vi "Teleop.vi"(10 "Match Info":T1={"Autonomous Elapsed Seconds"=0.0, "TeleOp Elapsed Seconds"=0.0, "Disabled Elapsed Seconds"=0.0, "Visited Autonomous"=FALSE, "Visited TeleOp"=FALSE, "Visited Disabled"=FALSE, "Autonomous Settings"={"Autonomous Style"=enum."Independent", "VI Refnum"=refnum}}, 11 "Call Context":T2) -> ()   [LabVIEW 2014]
doc: "This VI is called for each TeleOp packet received from the DS where the robot is not disabled. It is often used to read from the joysticks and update I/O or to update setpoints for timed control loops. It should complete and return within 20 milliseconds or it may miss DS packets."
uses:
  <vilib>/Rock Robotics/WPI/DriverStation/WPI_DriverStationDerivedRobotMode.ctl
  <vilib>/Rock Robotics/WPI/DriverStation/WPI_DriverStationMatch Info.ctl
  <vilib>/Rock Robotics/WPI/RobotDrive/WPI_RobotDriveGetSetRefNum.vi
  <vilib>/Rock Robotics/WPI/Joystick/WPI_JoystickGetSetRefNum.vi
  Robot Global Data.vi
  <vilib>/Rock Robotics/Network Tables/SD Write Boolean Array.vi
  <vilib>/Rock Robotics/Network Tables/SD Write Numeric Array.vi
  <vilib>/Rock Robotics/Network Tables/SD Read Number.vi
  <vilib>/Rock Robotics/Network Tables/SD Write Boolean.vi
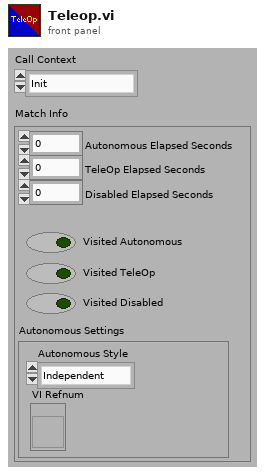
[diagram p1: front panel]
types:
  T1 = typedef "WPI_DriverStationMatch Info.ctl" = cluster{"Autonomous Elapsed Seconds":dbl, "TeleOp Elapsed Seconds":dbl, "Disabled Elapsed Seconds":dbl, "Visited Autonomous":bool, "Visited TeleOp":bool, "Visited Disabled":bool, "Autonomous Settings":cluster{"Autonomous Style":enum16{"Iterative", "Independent"}, "VI Refnum":refnum<vi>}}
  T2 = typedef "WPI_DriverStationDerivedRobotMode.ctl" = enum16{"Init", "Execute", "Stop"}
  T3 = typedef "WPI_JoystickDevRef.ctl" = cluster{"Device":T4}
  T4 = typedef "WPI_JoystickDeviceEnum.ctl" = enum16{"USB 0", "USB 1", "USB 2", "USB 3", "USB 4", "USB 5"}
  T5 = cluster{"POVs[0]":i16, "POVs[1]":i16, "POVs[2]":i16, "POVs[3]":i16, "POVs[4]":i16, "POVs[5]":i16, "POVs[6]":i16, "POVs[7]":i16, "POVs[8]":i16}
  T6 = cluster{"TopLeft":bool, "TopCenter":bool, "TopRight":bool, "MiddleRight":bool, "MiddleLeft":bool, "MiddleCenter":bool, "BottomRight":bool, "BottomLeft":bool, "BottomCenter":bool, "Top":bool, "Middle":bool, "Bottom":bool, "Left":bool, "Center":bool, "Right":bool}
  T7 = cluster{"Axes[0]":dbl, "Axes[1]":dbl, "Axes[2]":dbl, "Axes[3]":dbl, "Axes[4]":dbl, "Axes[5]":dbl, "Axes[6]":dbl, "Axes[7]":dbl, "Axes[8]":dbl}
  T8 = cluster{"Buttons[0]":bool, "Buttons[1]":bool, "Buttons[2]":bool, "Buttons[3]":bool, "Buttons[4]":bool, "Buttons[5]":bool, "Buttons[6]":bool, "Buttons[7]":bool, "Buttons[8]":bool, "Buttons[9]":bool, "Buttons[10]":bool, "Buttons[11]":bool, "Buttons[12]":bool, "Buttons[13]":bool, "Buttons[14]":bool, "Buttons[15]":bool}
  T9 = cluster{"Buttons[0]":bool, "Buttons[1]":bool, "Buttons[2]":bool, "Buttons[3]":bool, "Buttons[4]":bool, "Buttons[5]":bool, "Buttons[6]":bool, "Buttons[7]":bool, "Buttons[8]":bool}
  T10 = typedef "WPI_RobotDriveDevRef.ctl" = cluster{"DevStatus":errorcluster, "Motors[]":T11[], "Square Inputs":bool, "Max Output":dbl}
  T11 = typedef "WPI_MotorControlDeviceRef.ctl" = cluster{"DeviceStatus":errorcluster, "Type":T12, "PWM":cluster{"Controller":T13, "PWM Channel":T14, "DeadBand":T15}, "CAN":cluster{"Device Number":u8, "Control Mode":T16, "Semaphore":T17, "Max Vout":dbl, "TalonSRX Control Mode":T18}, "Invert":bool, "TransformRef":T19, "InvTransformRef":T19}
  T12 = typedef "WPI_MotorControlType.ctl" = enum16{"PWM", "CAN", "CANTalonSRX"}
  T13 = typedef "FPGA_TypedefDigitalModule.ctl" = enum16{"Controller 1"}
  T14 = typedef "FPGA_DIOPWMChannel.ctl" = enum8{"PWM 0", "PWM 1", "PWM 2", "PWM 3", "PWM 4", "PWM 5", "PWM 6", "PWM 7", "PWM 8", "PWM 9", "PWM MXP 0", "PWM MXP 1", "PWM MXP 2", "PWM MXP 3", "PWM MXP 4", "PWM MXP 5", "PWM MXP 6", "PWM MXP 7", "PWM MXP 8", "PWM MXP 9", "Invalid"}
  T15 = typedef "WPI_PWMDeadband.ctl" = cluster{"Name":string, "maxPositivePwm":i32, "minPositivePwm":i32, "centerPwm":i32, "maxNegativePwm":i32, "minNegativePwm":i32, "angularRange":u16}
  T16 = typedef "WPI_CANJaguar_ControlMode.ctl" = enum8{"Percent VBus", "Current", "Speed", "Position", "Voltage"}
  T17 = typedef "Semaphore RefNum" = refnum<k1>
  T18 = typedef "WPI_CANTalonSRX_APIControlMode.ctl" = enum8{"Percent VBus", "Speed", "Position", "Slave", "Unchanged / Invalid"}
  T19 = typedef "WPI_PWMTransform_ConPane.ctl" = refnum<vi>
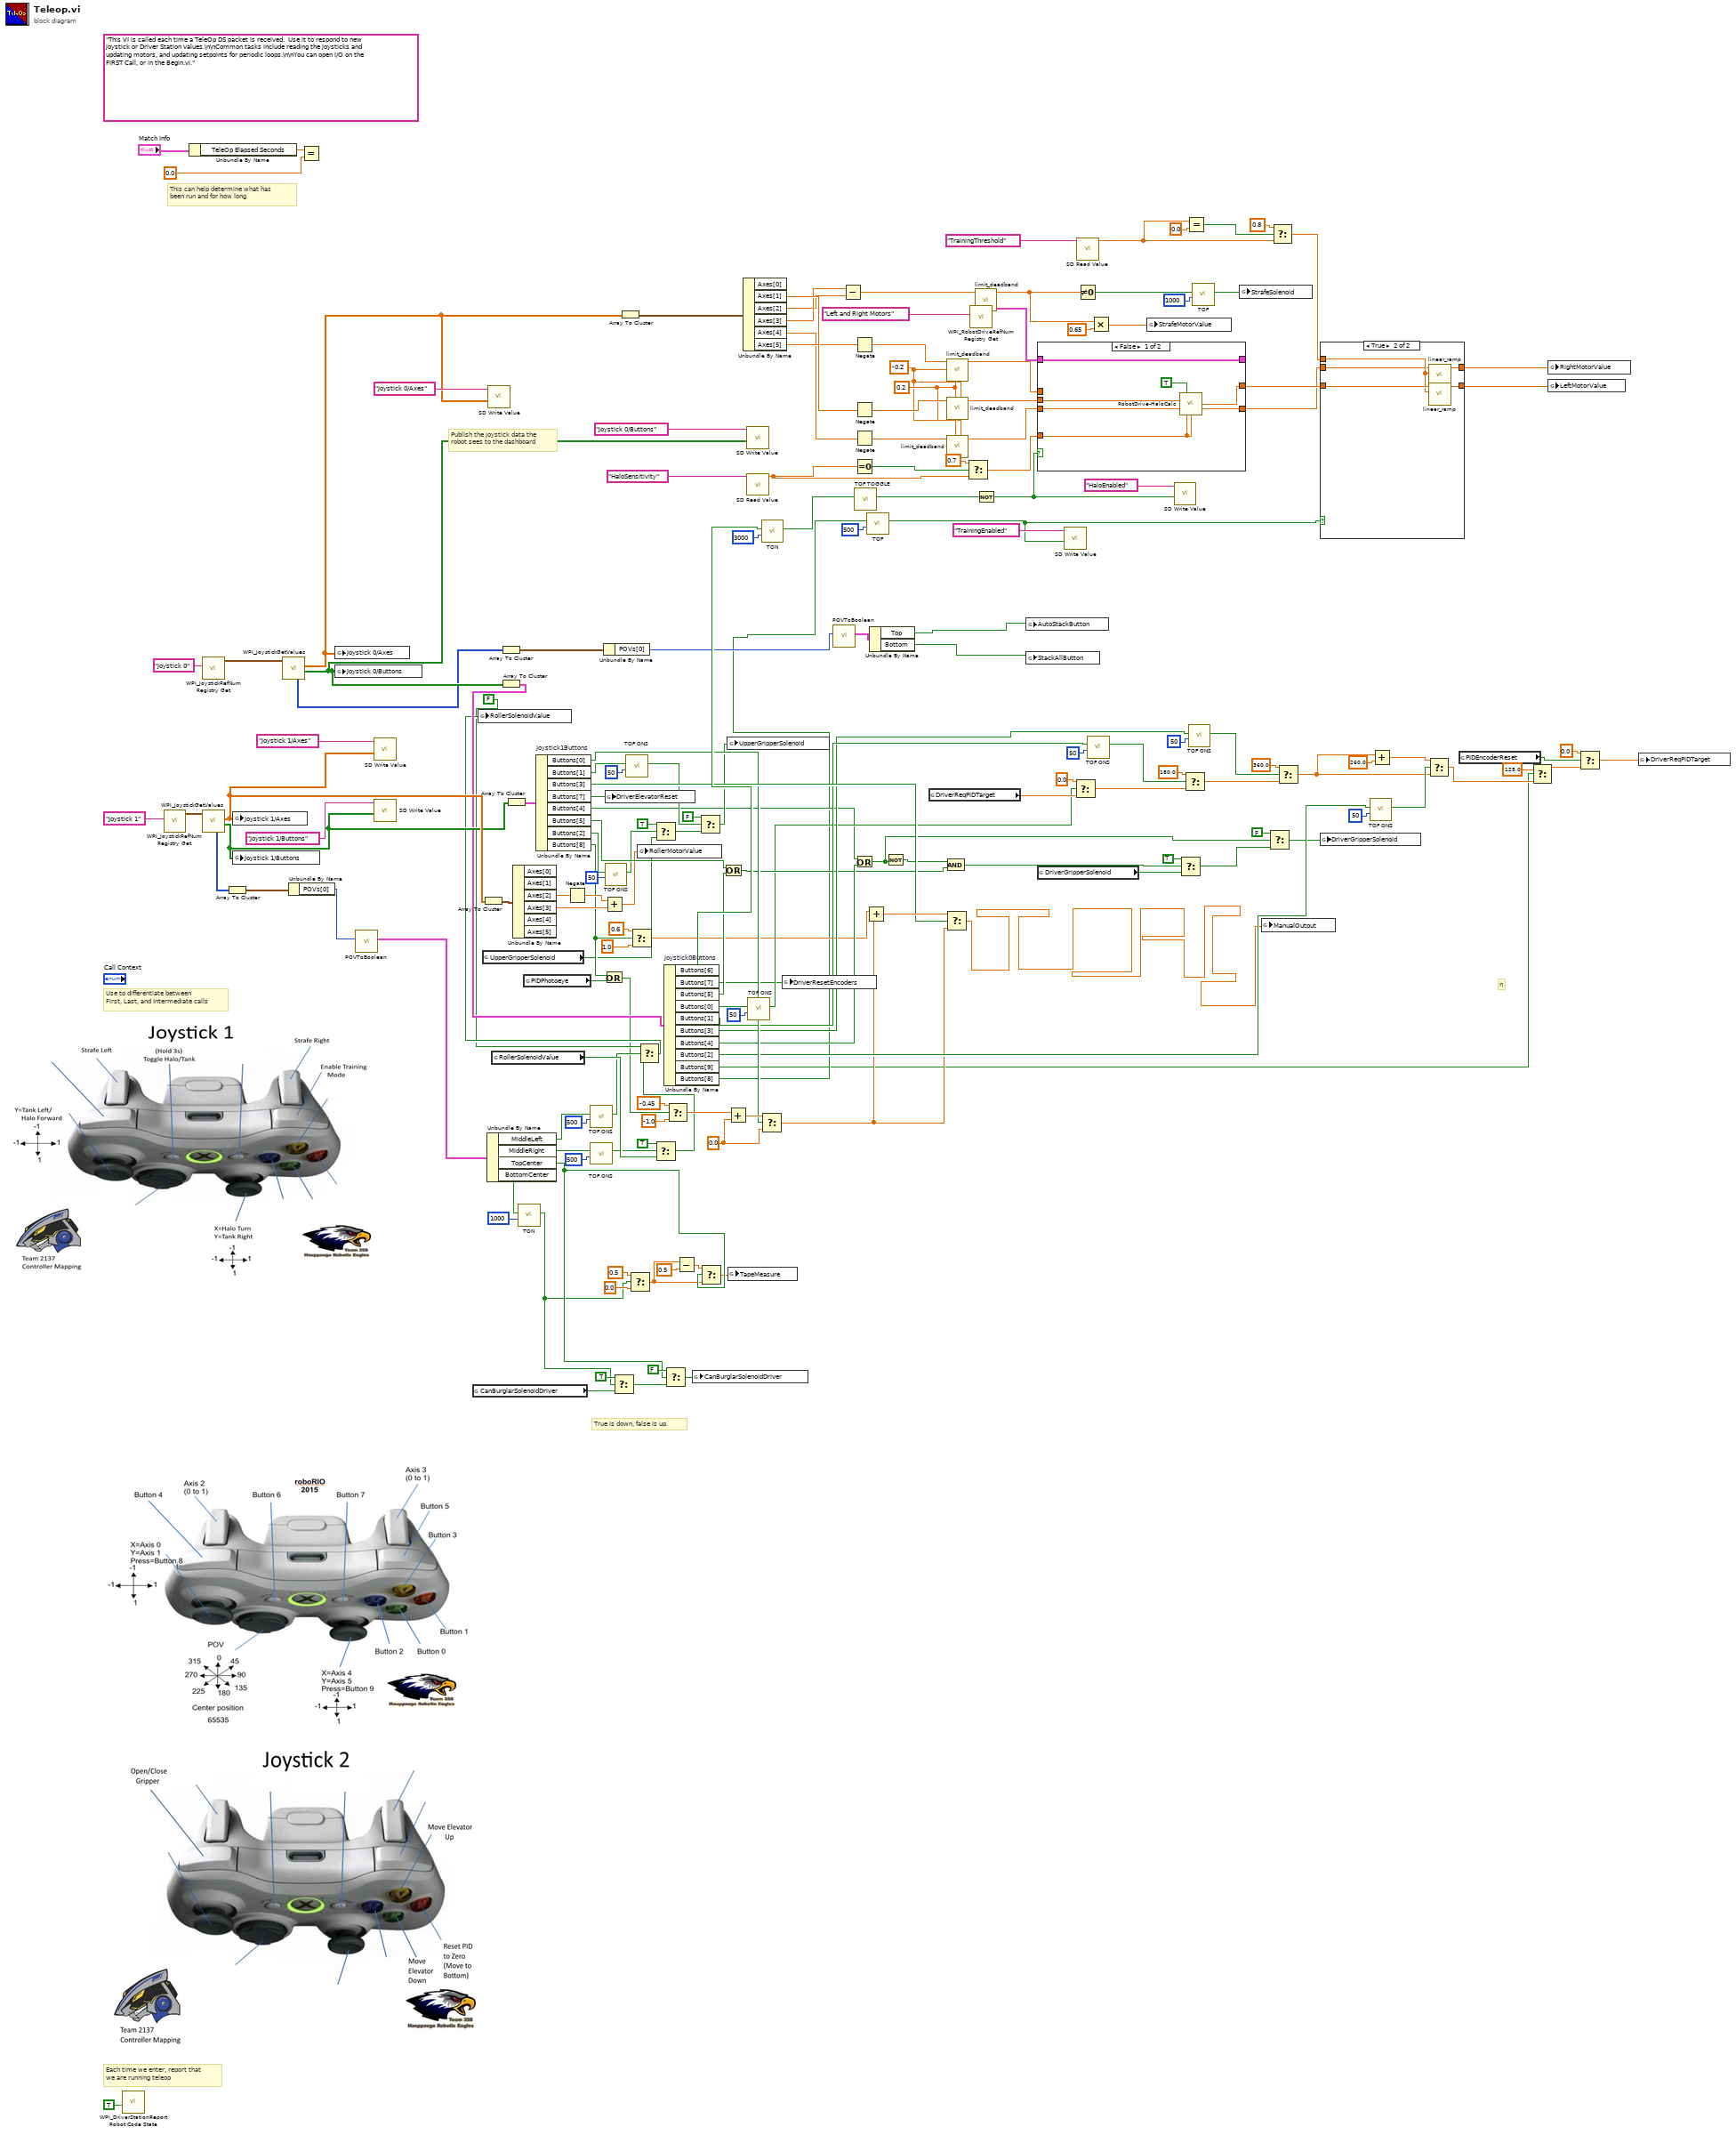
[diagram p0: block diagram]
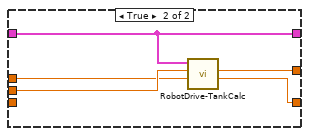
[diagram p3: hidden frame]
diagram:
  w78 = -0.2
  w79 = 0.2
  w141 = 0.0
  (unwired) "This VI is called each time a TeleOp DS packet is received.  Use it to respond to new joystick or Driver Station values.\n\nCommon tasks include reading the joysticks and updating motors, and updating setpoints for periodic loops.\n\nYou can open I/O on the FIRST Call, or in the Begin.vi."
  # "n"
  # "True is down, false is up."
  # "Publish the joystick data the\nrobot sees to the dashboard"
  # "Each time we enter, report that\nwe are running teleop"
  # "Use to differentiate between\nFirst, Last, and Intermediate calls"
  # "This can help determine what has\nbeen run and for how long"
  n1 = call <vilib>:"WPI_DriverStationReport Robot Code State.vi"("TeleOp"=TRUE ("Autonomous")) -> ()  [unwired: 10 in, 1 out]
  n2 = call <vilib>:"WPI_JoystickRefNum Registry Get.vi"("refnum name"="Joystick 1") -> ("JoystickDevRef"=w152:T3)  [unwired: 1 in, 9 out]
  n3 = Unbundle By Name("Match Info") -> ("TeleOp Elapsed Seconds"=w144:dbl)
  n4 = call <vilib>:"WPI_JoystickRefNum Registry Get.vi"("refnum name"="Joystick 0") -> ("JoystickDevRef"=w174:T3)  [unwired: 1 in, 9 out]
  n5 = call <vilib>:"WPI_JoystickGetValues.vi"("JoystickDevRef"=w152) -> ("Buttons"=w147:bool[], "Axes"=w148:dbl[], "POVs"=w58:i16[])  [unwired: 6 in, 2 out]
  n6 = Array To Cluster(array=w58) -> (cluster=w57:T5)
  n7 = global write "Robot Global Data.vi" "Joystick 1/Axes"(w148) -> ()
  n8 = global write "Robot Global Data.vi" "Joystick 1/Buttons"(w147) -> ()
  n9 = call <vilib>:"WPI_JoystickGetValues.vi"("JoystickDevRef"=w174) -> ("Buttons"=w145:bool[], "Axes"=w146:dbl[], "POVs"=w102:i16[])  [unwired: 6 in, 2 out]
  n10 = Unbundle By Name(w57) -> ("POVs[0]"=w56:i16)
  n11 = Equal?(x=w144, y=0.0) -> ()  [unwired: 1 out]
  n12 = global write "Robot Global Data.vi" "Joystick 0/Axes"(w146) -> ()
  n13 = global write "Robot Global Data.vi" "Joystick 0/Buttons"(w145) -> ()
  n14 = call "POVToBoolean.vi"("Input"=w56) -> ("Output"=w55:T6)  [unwired: 10 in]
  n15 = call-poly <vilib>:"SD Write Value.vi"("Numeric Array"=w148, "Name"="Joystick 1/Axes") -> ()  [unwired: 8 in, 2 out]
  n16 = call-poly <vilib>:"SD Write Value.vi"("Boolean Array"=w147, "Name"="Joystick 1/Buttons") -> ()  [unwired: 8 in, 2 out]
  n17 = global read "Robot Global Data.vi" "CanBurglarSolenoidDriver"() -> (w19:bool)
  n18 = Array To Cluster(array=w148) -> (cluster=w149:T7)
  n19 = global read "Robot Global Data.vi" "UpperGripperSolenoid"() -> (w22:bool)
  n20 = Unbundle By Name(w55) -> ("MiddleLeft"=w53:bool, "MiddleRight"=w54:bool, "TopCenter"=w16:bool, "BottomCenter"=w2:bool)
  n21 = call-poly <vilib>:"SD Write Value.vi"("Numeric Array"=w146, "Name"="Joystick 0/Axes") -> ()  [unwired: 8 in, 2 out]
  n22 = global read "Robot Global Data.vi" "RollerSolenoidValue"() -> (w50:bool)
  n23 = Array To Cluster(array=w102) -> (cluster=w103:T5)
  n24 = Array To Cluster(array=w145) -> (cluster=w77:T8)
  n25 = Array To Cluster(array=w147) -> (cluster=w142:T9)
  n26 = Unbundle By Name(w149) -> ("Axes[2]"=w63:dbl, "Axes[3]"=w44:dbl)  [unwired: 4 out]
  n27 = call "TON.vi"("Delay (ms)"=u32 1000, "Input"=w2) -> ("Output"=w3:bool)  [unwired: 9 in]
  n28 = global read "Robot Global Data.vi" "PIDPhotoeye"() -> (w89:bool)
  n29 = Unbundle By Name "Joystick1Buttons"(w142) -> ("Buttons[0]"=w128:bool, "Buttons[1]"=w35:bool, "Buttons[3]"=w129:bool, "Buttons[7]"=w107:bool, "Buttons[4]"=w27:bool, "Buttons[5]"=w75:bool, "Buttons[2]"=w33:bool, "Buttons[8]"=w38:bool)
  n30 = Negate(x=w63) -> (-x=w45:dbl)
  n31 = call "TOF ONS.vi"("Delay (ms)"=u32 500, "Input"=w53) -> ("Output"=w46:bool)  [unwired: 9 in]
  n32 = call "TOF ONS.vi"("Delay (ms)"=u32 500, "Input"=w54) -> ("Output"=w48:bool)  [unwired: 9 in]
  n33 = Unbundle By Name(w103) -> ("POVs[0]"=w42:i16)
  n34 = Add(x=w45, y=w44) -> (x+y=w62:dbl)
  n35 = Or(x=w38, y=w89) -> (x .or. y?=w43:bool)
  n36 = global write "Robot Global Data.vi" "DriverElevatorReset"(w107) -> ()
  n37 = call "TOF ONS.vi"("Delay (ms)"=u32 50, "Input"=w33) -> ("Output"=w28:bool)  [unwired: 9 in]
  n38 = Select(t=TRUE, s=w3, f=w19) -> (s? t:f=w20:bool)
  n39 = Array To Cluster(array=w146) -> (cluster=w170:T7)
  n40 = call "TOF ONS.vi"("Delay (ms)"=u32 50, "Input"=w35) -> ("Output"=w30:bool)  [unwired: 9 in]
  n41 = Select(t=0.5 ("y"), s=w3, f=0.0) -> (s? t:f=w10:dbl)
  n42 = Select(t=0.6, s=w38, f=1.0 ("x")) -> (s? t:f=w37:dbl)
  n43 = global write "Robot Global Data.vi" "RollerMotorValue"(w62) -> ()
  n44 = Select(t=TRUE, s=w28, f=w22) -> (s? t:f=w29:bool)
  n45 = Select(t=TRUE, s=w48, f=w50) -> (s? t:f=w51:bool)
  n46 = Select(t=FALSE, s=w46, f=w51) -> (s? t:f=w52:bool)
  n47 = global write "Robot Global Data.vi" "RollerSolenoidValue"(w52) -> ()
  n48 = Unbundle By Name "Joystick0Buttons"(w77) -> ("Buttons[6]"=w158:bool, "Buttons[7]"=w9:bool, "Buttons[5]"=w76:bool, "Buttons[0]"=w122:bool, "Buttons[1]"=w125:bool, "Buttons[3]"=w118:bool, "Buttons[4]"=w74:bool, "Buttons[2]"=w108:bool, "Buttons[9]"=w5:bool, "Buttons[8]"=w8:bool)
  n49 = Select(t=FALSE, s=w16, f=w20) -> (s? t:f=w21:bool)
  n50 = Select(t=-0.45, s=w43, f=-1.0 ("x")) -> (s? t:f=w86:dbl)
  n51 = Subtract(x=w10, y=0.5) -> (x-y=w14:dbl)
  n52 = global write "Robot Global Data.vi" "CanBurglarSolenoidDriver"(w21) -> ()
  n53 = Select(t=FALSE, s=w30, f=w29) -> (s? t:f=w31:bool)
  n54 = Select(t=w14, s=w16, f=w10) -> (s? t:f=w15:dbl)
  n55 = Or(x=w75, y=w76) -> (x .or. y?=w67:bool)
  n56 = global write "Robot Global Data.vi" "UpperGripperSolenoid"(w31) -> ()
  n57 = Add(x=w86, y=w141) -> (x+y=w140:dbl)
  n58 = global write "Robot Global Data.vi" "TapeMeasure"(w15) -> ()
  n59 = Unbundle By Name(w170) -> ("Axes[1]"=w169:dbl, "Axes[2]"=w163:dbl, "Axes[3]"=w164:dbl, "Axes[4]"=w155:dbl, "Axes[5]"=w167:dbl)  [unwired: 1 out]
  n60 = call-poly <vilib>:"SD Write Value.vi"("Boolean Array"=w145, "Name"="Joystick 0/Buttons") -> ()  [unwired: 8 in, 2 out]
  n61 = call-poly <vilib>:"SD Read Value.vi"("Name"="HaloSensitivity") -> ("Numeric"=w99:dbl)  [unwired: 8 in, 2 out]
  n62 = call "TOF ONS.vi"("Delay (ms)"=u32 50, "Input"=w122) -> ("Output"=w61:bool)  [unwired: 9 in]
  n63 = Select(t=w140, s=w128, f=w141) -> (s? t:f=w65:dbl)
  n64 = call "TON.vi"("Delay (ms)"=u32 3000, "Input"=w158) -> ("Output"=w159:bool)  [unwired: 9 in]
  n65 = global write "Robot Global Data.vi" "DriverResetEncoders"(w9) -> ()
  n66 = call "POVToBoolean.vi"("Input"=w42) -> ("Output"=w41:T6)  [unwired: 10 in]
  n67 = Subtract(x=w164, y=w163) -> (x-y=w165:dbl)
  n68 = Negate(x=w167) -> (-x=w166:dbl)
  n69 = Negate(x=w169) -> (-x=w168:dbl)
  n70 = Negate(x=w155) -> (-x=w156:dbl)
  n71 = Equal To 0?(x=w99) -> (x = 0?=w101:bool)
  n72 = Or(x=w27, y=w74) -> (x .or. y?=w36:bool)
  n73 = call "TOF TOGGLE.vi"("Input"=w159) -> ("Output"=w130:bool)  [unwired: 10 in]
  n74 = Add(x=w37, y=w65) -> (x+y=w139:dbl)
  n75 = call "TOF.vi"("Delay (ms)"=u32 500, "Input"=w8) -> ("Output"=w91:bool)  [unwired: 9 in]
  n76 = Unbundle By Name(w41) -> ("Top"=w25:bool, "Bottom"=w24:bool)
  n77 = Not(x=w36) -> (.not. x?=w66:bool)
  n78 = global read "Robot Global Data.vi" "DriverReqPIDTarget"() -> (w90:dbl)
  n79 = Select(t=w139, s=w129, f=w65) -> (s? t:f=w64:dbl)
  n80 = call "limit_deadband.vi"("lower limit"=w78, "upper limit"=w79, "Val"=w166) -> ("Val Out"=w160:dbl)  [unwired: 8 in]
  n81 = call "limit_deadband.vi"("lower limit"=w78, "upper limit"=w79, "Val"=w168) -> ("Val Out"=w161:dbl)  [unwired: 8 in]
  n82 = call "limit_deadband.vi"("lower limit"=w78, "upper limit"=w79, "Val"=w156) -> ("Val Out"=w154:dbl)  [unwired: 8 in]
  n83 = Compound Arithmetic op=AND(w66, w67) -> (w73:bool)
  n84 = Select(t=0.7, s=w101, f=w99) -> (s? t:f=w98:dbl)
  n85 = call <vilib>:"WPI_RobotDriveRefNum Registry Get.vi"("refnum name"="Left and Right Motors") -> ("RobotDriveDevRef"=w162:T10)  [unwired: 1 in, 9 out]
  n86 = call "limit_deadband.vi"("Val"=w165) -> ("Val Out"=w80:dbl)  [unwired: 10 in]
  n87 = Not(x=w130) -> (.not. x?=w114:bool)
  n88 = global write "Robot Global Data.vi" "AutoStackButton"(w25) -> ()
  n89 = global write "Robot Global Data.vi" "StackAllButton"(w24) -> ()
  n90 = case shown="False" w114 {
    tunnel: w162 -> [w181 w185]
    tunnel: [w184 w189] -> w136
    tunnel: [w183 w188] -> w133
    tunnel: w161 -> [w182 w187]
    tunnel: w160 -> [_ w186]
    tunnel: w98 -> [w178 _]
    tunnel: [w181 w185] -> _
    tunnel: w154 -> [w179 _]
    frame False {
      n91 = call "RobotDrive-HaloCalc.vi"("QwikTurnButton"=TRUE, "Left axis value"=w182, "Right axis value"=w179, "Sensitivity"=w178, "QuikTurn Sensitivity"=w178) -> ("Left Output"=w184:dbl, "Right Output"=w183:dbl)  [unwired: 9 in]
    }
    frame True {
      n92 = call "RobotDrive-TankCalc.vi"("Right axis value"=w186, "Left axis value"=w187, "RobotDriveDevRef"=w185) -> ("Right motor value"=w188:dbl, "Left motor value"=w189:dbl)  [unwired: 7 in]
    }
  }
  n93 = global read "Robot Global Data.vi" "DriverGripperSolenoid"() -> (w72:bool)
  n94 = call-poly <vilib>:"SD Write Value.vi"("Boolean"=w91, "Name"="TrainingEnabled") -> ()  [unwired: 8 in, 2 out]
  n95 = Select(t=0.0, s=w61, f=w90) -> (s? t:f=w126:dbl)
  n96 = call-poly <vilib>:"SD Read Value.vi"("Name"="TrainingThreshold") -> ("Numeric"=w94:dbl)  [unwired: 8 in, 2 out]
  n97 = Not Equal To 0?(x=w80) -> (x != 0?=w83:bool)
  n98 = call "TOF ONS.vi"("Delay (ms)"=u32 50, "Input"=w125) -> ("Output"=w123:bool)  [unwired: 9 in]
  n99 = Multiply(x=w80, y=0.65) -> (x*y=w85:dbl)
  n100 = global write "Robot Global Data.vi" "StrafeMotorValue"(w85) -> ()
  n101 = call-poly <vilib>:"SD Write Value.vi"("Boolean"=w114, "Name"="HaloEnabled") -> ()  [unwired: 8 in, 2 out]
  n102 = Select(t=TRUE, s=w73, f=w72) -> (s? t:f=w70:bool)
  n103 = Select(t=180.0, s=w123, f=w126) -> (s? t:f=w117:dbl)
  n104 = Equal?(x=w94, y=0.0) -> (x = y?=w96:bool)
  n105 = call "TOF ONS.vi"("Delay (ms)"=u32 50, "Input"=w118) -> ("Output"=w115:bool)  [unwired: 9 in]
  n106 = call "TOF.vi"("Delay (ms)"=u32 1000, "Input"=w83) -> ("Output"=w81:bool)  [unwired: 9 in]
  n107 = global write "Robot Global Data.vi" "StrafeSolenoid"(w81) -> ()
  n108 = global write "Robot Global Data.vi" "ManualOutput"(w64) -> ()
  n109 = Select(t=FALSE, s=w36, f=w70) -> (s? t:f=w68:bool)
  n110 = Select(t=0.8, s=w96, f=w94) -> (s? t:f=w93:dbl)
  n111 = Select(t=360.0, s=w115, f=w117) -> (s? t:f=w110:dbl)
  n112 = case shown="True" w91 {
    tunnel: [w191 w195] -> w135
    tunnel: w136 -> [w191 w196]
    tunnel: [w190 w192] -> w134
    tunnel: w133 -> [w190 w193]
    tunnel: w93 -> [_ w194]
    frame False {
    }
    frame True {
      n113 = call "linear_ramp.vi"("filter const (dx/dt)"=w194, "input"=w193) -> ("output"=w192:dbl)  [unwired: 9 in]
      n114 = call "linear_ramp.vi"("filter const (dx/dt)"=w194, "input"=w196) -> ("output"=w195:dbl)  [unwired: 9 in]
    }
  }
  n115 = global write "Robot Global Data.vi" "DriverGripperSolenoid"(w68) -> ()
  n116 = call "TOF ONS.vi"("Delay (ms)"=u32 50, "Input"=w108) -> ("Output"=w112:bool)  [unwired: 9 in]
  n117 = Add(x=w110, y=260.0) -> (x+y=w111:dbl)
  n118 = Select(t=w111, s=w112, f=w110) -> (s? t:f=w6:dbl)
  n119 = global read "Robot Global Data.vi" "PIDEncoderReset"() -> (w105:bool)
  n120 = Select(t=125.0, s=w5, f=w6) -> (s? t:f=w7:dbl)
  n121 = global write "Robot Global Data.vi" "RightMotorValue"(w134) -> ()
  n122 = global write "Robot Global Data.vi" "LeftMotorValue"(w135) -> ()
  n123 = Select(t=0.0, s=w105, f=w7) -> (s? t:f=w106:dbl)
  n124 = global write "Robot Global Data.vi" "DriverReqPIDTarget"(w106) -> ()
